vi "ConvertJsonToUML.vi"(9 "JSON":string) -> (1 "UML":string, 2 "ObjectsS":T1(array[cluster]))   [LabVIEW 2021, in "TAF Proj Document Type.lvlib" / "TAFConfiguration.lvclass"]
uses:
  <vilib>/Wovalab/AntiDoc/Document Type/Add-ons/LabVIEW TAF Project/TAFConfiguration/TAFConfiguration.lvclass
  382281d9-785c-4807-b68a-e5478ce20f5e.vi
  <vilib>/JDP Science/JSONtext/JSON text to Variant.vi
  <vilib>/JDP Science/JSONtext/LVClass Serializer/JSONtext LVClass Serializer.lvclass
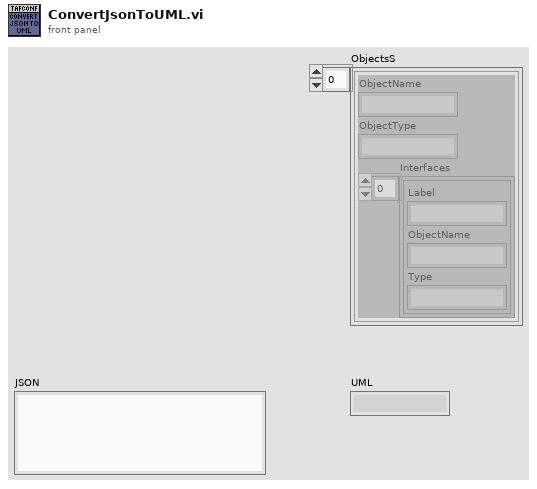
[diagram p1: front panel]
types:
  T1 = cluster{"ObjectName":string, "ObjectType":string, "Interfaces":cluster{"Label":string, "ObjectName":string, "Type":string}[]}[]
  T2 = cluster{"Objects":cluster{"ObjectName":string, "ObjectType":string, "Interfaces":cluster{"Label":string, "ObjectName":string, "Type":string}[]}[]}
  T3 = cluster{"Label":string, "ObjectName":string, "Type":string}[]
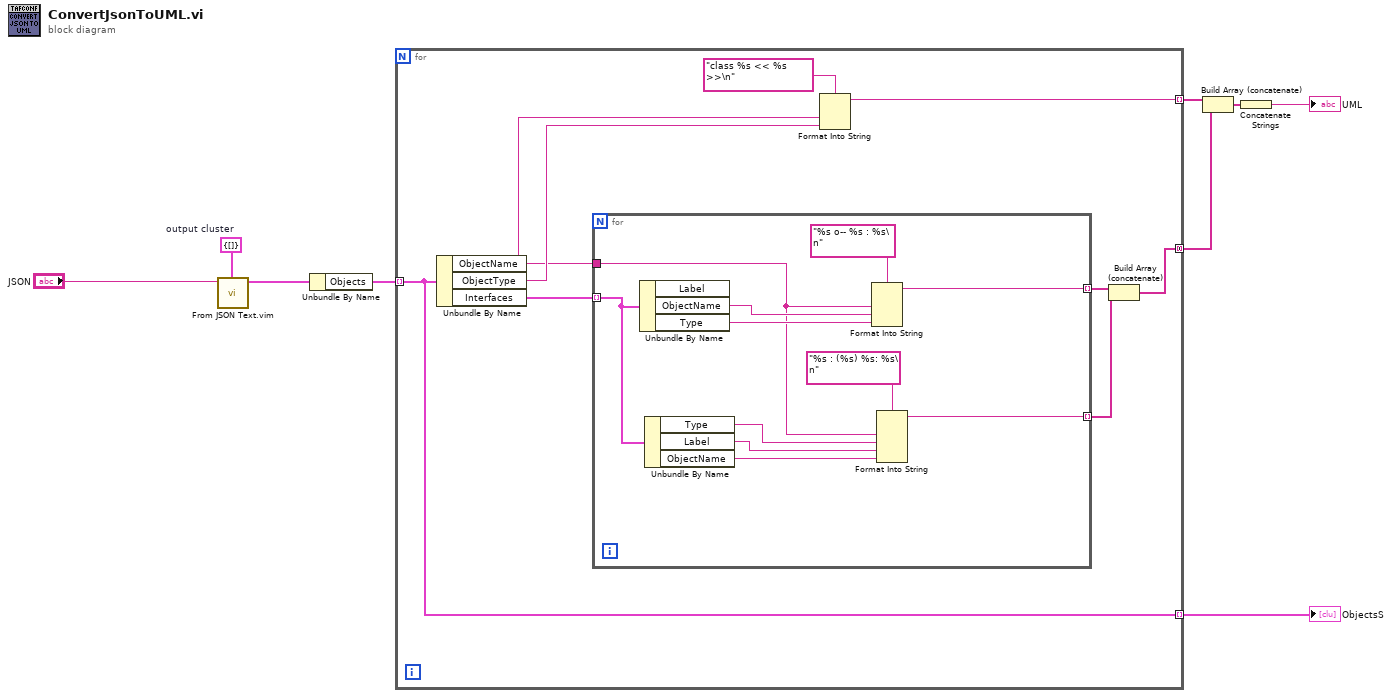
[diagram p0: block diagram]
diagram:
  w6 = T2 {"Objects"=[]}  # output cluster
  n1 = call "From JSON Text.vim"("Data Type and Default Value"=w6, "JSON"="JSON") -> ("Data out"=w7:T2)  [unwired: 8 in, 1 out]
  n2 = Unbundle By Name(w7) -> ("Objects"=w5:T1)
  n3 = for {
    tunnel: w5 -> [w10] mode=indexing
    tunnel: [w15] -> w4 mode=indexing
    tunnel: [w12] -> w3 mode=concatenating
    tunnel: [w10] -> w1 mode=indexing
    n4 = Unbundle By Name(w10) -> ("ObjectName"=w14:string, "ObjectType"=w16:string, "Interfaces"=w18:T3)
    n5 = for {
      tunnel: w18 -> [w24] mode=indexing
      tunnel: w14 -> [w22]
      tunnel: [w27] -> w13 mode=indexing
      tunnel: [w23] -> w11 mode=indexing
      n6 = Unbundle By Name(w24) -> ("ObjectName"=w28:string, "Type"=w26:string)  [unwired: 1 out]
      n7 = Unbundle By Name(w24) -> ("Type"=w21:string, "Label"=w19:string, "ObjectName"=w20:string)
      n8 = Format Into String(format string="%s o-- %s : %s\n", w22, w28, w26) -> (resulting string=w27:string)  [unwired: 2 in, 1 out]
      n9 = Format Into String(format string="%s : (%s) %s: %s\n", w22, w21, w19, w20) -> (resulting string=w23:string)  [unwired: 2 in, 1 out]
    }
    n10 = Format Into String(format string="class %s << %s  >>\n", w14, w16) -> (resulting string=w15:string)  [unwired: 2 in, 1 out]
    n11 = Build Array (concatenate)(w13, w11) -> (w12:string[])
  }
  "ObjectsS" <- w1
  n12 = Build Array (concatenate)(w4, w3) -> (w2:string[])
  n13 = Concatenate Strings(w2) -> (→"UML":string)
